vi "E441X_PM_Generate_Inst_Error.vi"(0 "VISA session":refnum<visa-resource-name>, 5 "Error State (F: Off)":bool, 7 "Code (0 - No error)":i32 format="%.0x", 11 "error in (no error)":errorcluster {"code" format="%.0x"}) -> (4 "dup VISA session":refnum<visa-resource-name>, 15 "error out":errorcluster {"code" format="%.0x"})   [LabVIEW 2015]
doc: "This VI generates the error cluster with Error Code as code and chain of VI as source. The source does not include the name of this VI."
panel:
  # "On"
  # "Off"
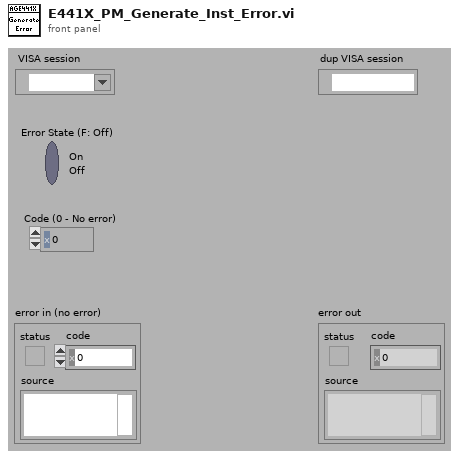
[diagram p1: front panel]
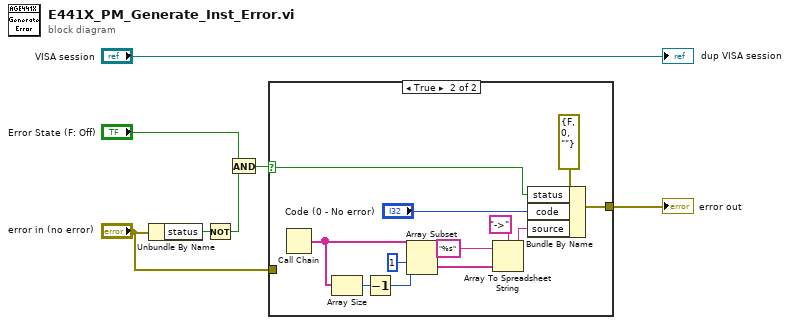
[diagram p0: block diagram]
diagram:
  n1 = Unbundle By Name("error in (no error)") -> ("status"=w2:bool)
  n2 = Not(x=w2) -> (.not. x?=w7:bool)
  n3 = And(x="Error State (F: Off)", y=w7) -> (x .and. y?=w5:bool)
  n4 = case shown="True" w5 {
    selector: w5 -> [_ w10]
    tunnel: [w8 w11] -> w3
    tunnel: "error in (no error)" -> [w8 _]
    frame False {
    }
    frame True {
      n5 = Call Chain() -> (call chain=w19:string[])
      n6 = Array Size(array=w19) -> (size(s)=w18:i32)
      n7 = Decrement(x=w18) -> (x-1=w17:i32)
      n8 = Array Subset(array=w19, index=1 ("Array Index"), length=w17) -> (w9:string[])
      n9 = Array To Spreadsheet String(delimiter (Tab)="->", array=w9, 3:"%s" ("format string")) -> (spreadsheet string=w12:string)
      n10 = Bundle By Name(cluster=errorcluster {"status"=FALSE, "code"=0, "source"=""} ("Error Out"), "status"=w10, "code"="Code (0 - No error)", "source"=w12) -> (w11:errorcluster)
    }
  }
  "error out" <- w3
  "dup VISA session" <- "VISA session"
